vi "Read.vi"(8 "error in":errorcluster, 11 "Cycler Cluster - 24 Channel.lvclass":refnum<class "Cycler Cluster - 6 Channel.lvclass">) -> (0 "error out":errorcluster, 3 "output cluster":refnum<class "Cycler Cluster - 6 Channel.lvclass">)   [LabVIEW 2023, in "Cycler Cluster - 6 Channel.lvclass"]
uses:
  Cycler Cluster - 6 Channel.lvclass
  Cycler Cluster - 6 Channel.lvclass/Cycler Cluster - 6 Channel.ctl
  e05ba3c7-7c94-4426-80ba-5afd499af12c.vi
  110d711f-602d-45bb-9c3c-bc18ca51752e.vi
  a3c512e7-962e-4a93-8488-56a803890fdd.vi
  4f6d0910-25e4-400a-b4c5-092e8cc88d34.vi
  4448cff9-e18d-4a6b-945e-10b1e3fd2828.vi
  4a46be96-aeb5-43b7-9243-adca9a8444cf.vi
  27230f32-3038-432e-846c-8983fd03581f.vi
  e05ba3c7-7c94-4426-80ba-5afd499af12c.vi/c28b0ead-42ad-4072-80a2-aca7f2bd7ce3.vi
  e05ba3c7-7c94-4426-80ba-5afd499af12c.vi/219d0231-d98b-4193-b5cc-84f90e3c9091.vi
  110d711f-602d-45bb-9c3c-bc18ca51752e.vi/c28b0ead-42ad-4072-80a2-aca7f2bd7ce3.vi
  110d711f-602d-45bb-9c3c-bc18ca51752e.vi/219d0231-d98b-4193-b5cc-84f90e3c9091.vi
  a3c512e7-962e-4a93-8488-56a803890fdd.vi/c28b0ead-42ad-4072-80a2-aca7f2bd7ce3.vi
  a3c512e7-962e-4a93-8488-56a803890fdd.vi/219d0231-d98b-4193-b5cc-84f90e3c9091.vi
  4f6d0910-25e4-400a-b4c5-092e8cc88d34.vi/c28b0ead-42ad-4072-80a2-aca7f2bd7ce3.vi
  4f6d0910-25e4-400a-b4c5-092e8cc88d34.vi/219d0231-d98b-4193-b5cc-84f90e3c9091.vi
  4448cff9-e18d-4a6b-945e-10b1e3fd2828.vi/c28b0ead-42ad-4072-80a2-aca7f2bd7ce3.vi
  4448cff9-e18d-4a6b-945e-10b1e3fd2828.vi/219d0231-d98b-4193-b5cc-84f90e3c9091.vi
  4a46be96-aeb5-43b7-9243-adca9a8444cf.vi/c28b0ead-42ad-4072-80a2-aca7f2bd7ce3.vi
  4a46be96-aeb5-43b7-9243-adca9a8444cf.vi/219d0231-d98b-4193-b5cc-84f90e3c9091.vi
  27230f32-3038-432e-846c-8983fd03581f.vi/c28b0ead-42ad-4072-80a2-aca7f2bd7ce3.vi
  27230f32-3038-432e-846c-8983fd03581f.vi/219d0231-d98b-4193-b5cc-84f90e3c9091.vi
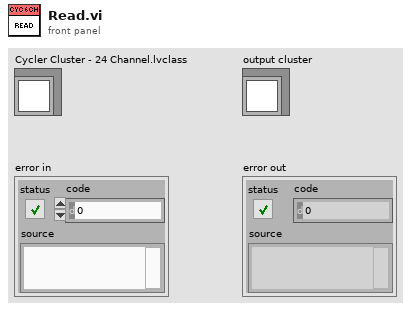
[diagram p1: front panel]
types:
  T1 = cluster{"OnOff.ACT":bool, "ErrorAcknowledge.ACT":bool, "IsoMeasurement.ACT":bool, "ParallelMode.ACT":bool}
  T2 = cluster{"ErrorAcknowledge.ch01.ACT":bool, "OutputEnable.ch01.ACT":bool, "ControlMode.ch01.CTL":u16, "Voltage.ch01.SP":dbl, "VoltageMIN.ch01.SP":dbl, "VoltageMAX.ch01.SP":dbl, "VoltageGrad.ch01.SP":dbl, "Current.ch01.SP":dbl, "CurrentMIN.ch01.SP":dbl, "CurrentMAX.ch01.SP":dbl, "CurrentGrad.ch01.SP":dbl, "Power.ch01.SP":dbl, "Power.ch01.SP":dbl, "Power.ch01.SP":dbl, "PowerGrad.ch01.SP":dbl, "ParameterSet.ch01.CTL":i32}
  T3 = cluster{"ErrorAcknowledge.ch02.ACT":bool, "OutputEnable.ch02.ACT":bool, "ControlMode.ch02.CTL":u16, "Voltage.ch02.SP":dbl, "VoltageMIN.ch02.SP":dbl, "VoltageMAX.ch02.SP":dbl, "VoltageGrad.ch02.SP":dbl, "Current.ch02.SP":dbl, "CurrentMIN.ch02.SP":dbl, "CurrentMAX.ch02.SP":dbl, "CurrentGrad.ch02.SP":dbl, "Power.ch02.SP":dbl, "PowerMIN.ch02.SP":dbl, "PowerMAX.ch02.SP":dbl, "PowerGrad.ch02.SP":dbl, "ParameterSet.ch02.CTL":i32}
  T4 = cluster{"ErrorAcknowledge.ch03.ACT":bool, "OutputEnable.ch03.ACT":bool, "ControlMode.ch03.CTL":u16, "Voltage.ch03.SP":dbl, "VoltageMIN.ch03.SP":dbl, "VoltageMAX.ch03.SP":dbl, "VoltageGrad.ch03.SP":dbl, "Current.ch03.SP":dbl, "CurrentMIN.ch03.SP":dbl, "CurrentMAX.ch03.SP":dbl, "CurrentGrad.ch03.SP":dbl, "Power.ch03.SP":dbl, "PowerMIN.ch03.SP":dbl, "PowerMAX.ch03.SP":dbl, "PowerGrad.ch03.SP":dbl, "ParameterSet.ch03.CTL":i32}
  T5 = cluster{"ErrorAcknowledge.ch04.ACT":bool, "OutputEnable.ch04.ACT":bool, "ControlMode.ch04.CTL":u16, "Voltage.ch04.SP":dbl, "VoltageMIN.ch04.SP":dbl, "VoltageMAX.ch04.SP":dbl, "VoltageGrad.ch04.SP":dbl, "Current.ch04.SP":dbl, "CurrentMIN.ch04.SP":dbl, "CurrentMAX.ch04.SP":dbl, "CurrentGrad.ch04.SP":dbl, "Power.ch04.SP":dbl, "PowerMIN.ch04.SP":dbl, "PowerMAX.ch04.SP":dbl, "PowerGrad.ch04.SP":dbl, "ParameterSet.ch04.CTL":i32}
  T6 = cluster{"ErrorAcknowledge.ch05.ACT":bool, "OutputEnable.ch05.ACT":bool, "ControlMode.ch05.CTL":u16, "Voltage.ch05.SP":dbl, "VoltageMIN.ch05.SP":dbl, "VoltageMAX.ch05.SP":dbl, "VoltageGrad.ch05.SP":dbl, "Current.ch05.SP":dbl, "CurrentMIN.ch05.SP":dbl, "CurrentMAX.ch05.SP":dbl, "CurrentGrad.ch05.SP":dbl, "Power.ch05.SP":dbl, "PowerMIN.ch05.SP":dbl, "PowerMAX.ch05.SP":dbl, "PowerGrad.ch05.SP":dbl, "ParameterSet.ch05.CTL":i32}
  T7 = cluster{"ErrorAcknowledge.ch06.ACT":bool, "OutputEnable.ch06.ACT":bool, "ControlMode.ch06.CTL":u16, "Voltage.ch06.SP":dbl, "VoltageMIN.ch06.SP":dbl, "VoltageMAX.ch06.SP":dbl, "VoltageGrad.ch06.SP":dbl, "Current.ch06.SP":dbl, "CurrentMIN.ch06.SP":dbl, "CurrentMAX.ch06.SP":dbl, "CurrentGrad.ch06.SP":dbl, "Power.ch06.SP":dbl, "PowerMIN.ch06.SP":dbl, "PowerMAX.ch06.SP":dbl, "PowerGrad.ch06.SP":dbl, "ParameterSet.ch06.CTL":i32}
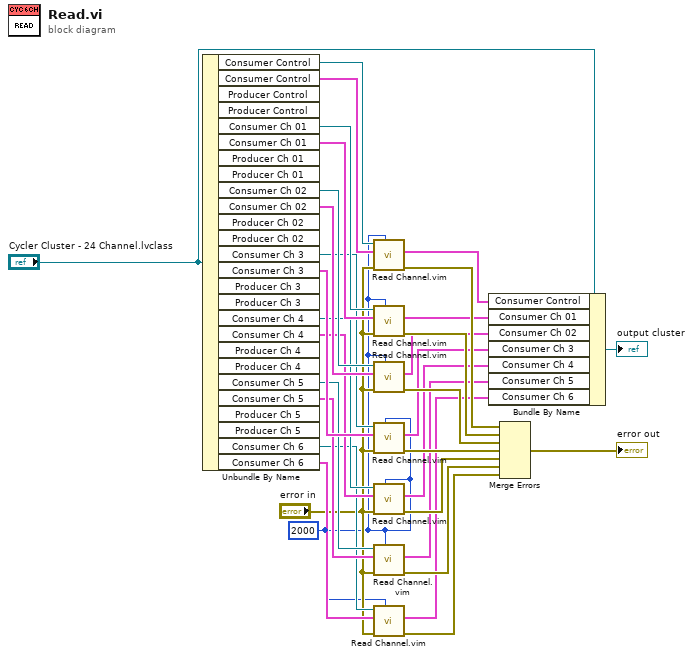
[diagram p0: block diagram]
diagram:
  w1 = 2000 ("Timeout (ms)")
  n1 = Unbundle By Name("Cycler Cluster - 24 Channel.lvclass") -> ("Consumer Control"=w24:refnum<k21>, "Consumer Control"=w23:T1, "Consumer Ch 01"=w22:refnum<k21>, "Consumer Ch 01"=w21:T2, "Consumer Ch 02"=w20:refnum<k21>, "Consumer Ch 02"=w19:T3, "Consumer Ch 3"=w18:refnum<k21>, "Consumer Ch 3"=w17:T4, "Consumer Ch 4"=w16:refnum<k21>, "Consumer Ch 4"=w15:T5, "Consumer Ch 5"=w14:refnum<k21>, "Consumer Ch 5"=w13:T6, "Consumer Ch 6"=w6:refnum<k21>, "Consumer Ch 6"=w5:T7)  [unwired: 12 out]
  n2 = call "Read Channel.vim"("Timeout (ms)"=w1, "error in"="error in", "Data in"=w23, "ADAS HIL Channel in"=w24) -> ("error out"=w32:errorcluster, "Data out"=w33:T1)  [unwired: 4 in, 2 out]
  n3 = call "Read Channel.vim"("Timeout (ms)"=w1, "error in"="error in", "Data in"=w21, "ADAS HIL Channel in"=w22) -> ("error out"=w31:errorcluster, "Data out"=w29:T2)  [unwired: 4 in, 2 out]
  n4 = call "Read Channel.vim"("Timeout (ms)"=w1, "error in"="error in", "Data in"=w19, "ADAS HIL Channel in"=w20) -> ("error out"=w28:errorcluster, "Data out"=w27:T3)  [unwired: 4 in, 2 out]
  n5 = call "Read Channel.vim"("Timeout (ms)"=w1, "error in"="error in", "Data in"=w17, "ADAS HIL Channel in"=w18) -> ("error out"=w12:errorcluster, "Data out"=w9:T4)  [unwired: 4 in, 2 out]
  n6 = call "Read Channel.vim"("Timeout (ms)"=w1, "error in"="error in", "Data in"=w15, "ADAS HIL Channel in"=w16) -> ("error out"=w11:errorcluster, "Data out"=w8:T5)  [unwired: 4 in, 2 out]
  n7 = call "Read Channel.vim"("Timeout (ms)"=w1, "error in"="error in", "Data in"=w13, "ADAS HIL Channel in"=w14) -> ("error out"=w10:errorcluster, "Data out"=w7:T6)  [unwired: 4 in, 2 out]
  n8 = call "Read Channel.vim"("Timeout (ms)"=w1, "error in"="error in", "Data in"=w5, "ADAS HIL Channel in"=w6) -> ("error out"=w2:errorcluster, "Data out"=w4:T7)  [unwired: 4 in, 2 out]
  n9 = Bundle By Name(cluster="Cycler Cluster - 24 Channel.lvclass", "Consumer Control"=w33, "Consumer Ch 01"=w29, "Consumer Ch 02"=w27, "Consumer Ch 3"=w9, "Consumer Ch 4"=w8, "Consumer Ch 5"=w7, "Consumer Ch 6"=w4) -> (→"output cluster":refnum<class "Cycler Cluster - 6 Channel.lvclass">)
  n10 = Merge Errors(w32, w31, w28, w12, w11, w10, w2) -> (→"error out":errorcluster)
